vi "Resolve Section Node Dependencies.vi"(8 "error in":errorcluster, 9 "Section Types":string[](array[string]), 10 "Section Clusters":refnum<vi>[](array[refnum]), 11 "Sections":refnum<k20>[](array[refnum])) -> (0 "error out":errorcluster, 1 "Section Types":string[](array[string]), 2 "Section Clusters":refnum<vi>[](array[refnum]), 3 "Sections":refnum<k20>[](array[refnum]))   [LabVIEW 2026, in "XML Parser.lvlib"]
uses:
  XML Parser.lvlib
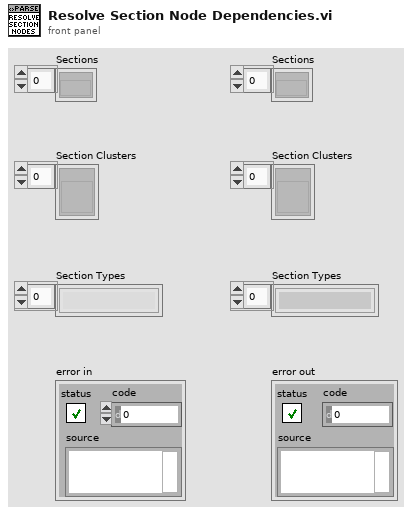
[diagram p1: front panel]
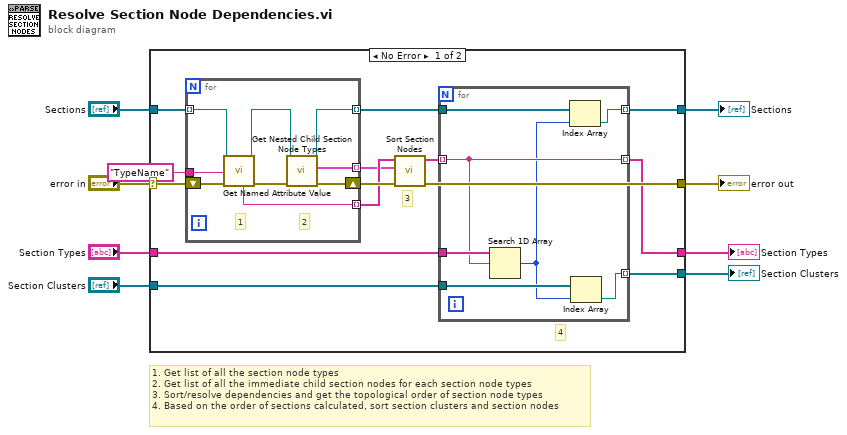
[diagram p0: block diagram]
diagram:
  # "1. Get list of all the section node types\n2. Get list of all the immediate child section nodes for each section node types\n3. Sort/resolve dependencies and get the topological order of section node types\n4. Based on the order of sections calculated, sort section clusters and section nodes"
  n1 = case shown="No Error" "error in" {
    selector: "error in" -> [w22 w42]
    tunnel: [w21 w42] -> w8
    tunnel: "Sections" -> [w19 w41]
    tunnel: [w10 w41] -> w5
    tunnel: "Section Types" -> [w15 w40]
    tunnel: [w14 w40] -> w3
    tunnel: "Section Clusters" -> [w13 w39]
    tunnel: [w12 w39] -> w1
    frame No Error {
      # "4"
      # "3"
      n2 = for {
        tunnel: w19 -> [w35] mode=indexing
        shift-right: [w36] -> w20
        shift-left: w22 -> [w38]
        tunnel: [w33] -> w11 mode=indexing
        tunnel: [w32] -> w17 mode=indexing
        tunnel: [w31] -> w18 mode=indexing
        tunnel: "TypeName" ("Attribute Name") -> [w30]
        # "2"
        # "1"
        n3 = call "Get Named Attribute Value.vi"("error in"=w38, "Attribute Name"=w30, "Node In"=w35) -> ("error out"=w37:errorcluster, "Node Out"=w34:refnum<k20>, "Attribute Value"=w31:string)  [unwired: 5 in, 1 out]
        n4 = call "Get Nested Child Section Node Types.vi"("error in"=w37, "Node"=w34) -> ("error out"=w36:errorcluster, "Nested Section Types"=w32:cluster{"Nested Section Types":string[]}, "Node"=w33:refnum<k20>)  [unwired: 7 in]
      }
      n5 = call "Sort Section Nodes.vi"("error in"=w20, "Nested Section Types"=w17, "Section TypeNames"=w18) -> ("error out"=w21:errorcluster, "Sorted Section TypeNames"=w16:string[])  [unwired: 7 in]
      n6 = for {
        tunnel: w16 -> [w28] mode=indexing
        tunnel: w15 -> [w29]
        tunnel: [w28] -> w14 mode=indexing
        tunnel: w13 -> [w27]
        tunnel: [w26] -> w12 mode=indexing
        tunnel: w11 -> [w25]
        tunnel: [w23] -> w10 mode=indexing
        n7 = Search 1D Array(1D array=w29, element=w28) -> (index of element=w24:i32)  [unwired: 1 in]
        n8 = Index Array(array=w25, index=w24) -> (element=w23:refnum<k20>)
        n9 = Index Array(array=w27, index=w24) -> (element=w26:refnum<vi>)
      }
    }
    frame Error {
    }
  }
  "error out" <- w8
  "Sections" <- w5
  "Section Types" <- w3
  "Section Clusters" <- w1
